vi "Read Data.vi"(8 "error in (no error)":errorcluster, 11 "WebSocket Data Handler Msg in":refnum<class "WebSocket Connection Handler Msg.lvclass">) -> (0 "error out":errorcluster, 2 "Data":string, 3 "WebSocket Data Handler Msg out":refnum<class "WebSocket Connection Handler Msg.lvclass">)   [LabVIEW 2016, in "WebSocket Actors.lvlib" / "WebSocket Connection Handler Msg.lvclass"]
uses:
  WebSocket Connection Handler Msg.lvclass
  WebSocket Connection Handler Msg.lvclass/WebSocket Connection Handler Msg.ctl
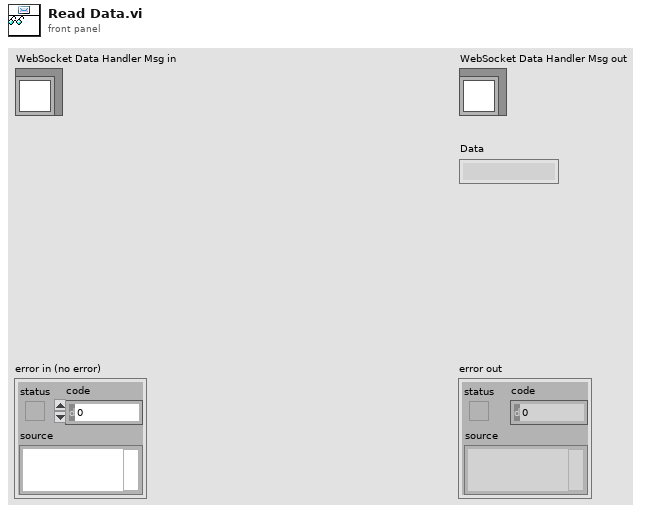
[diagram p1: front panel]
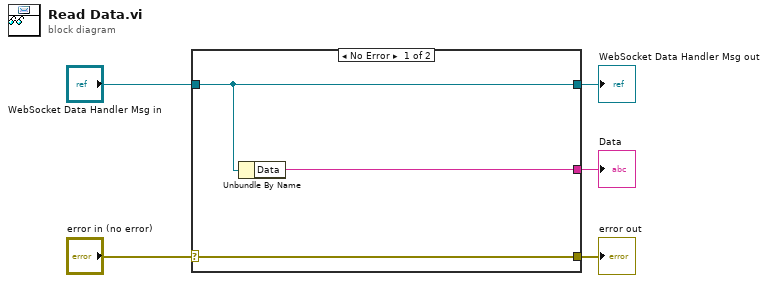
[diagram p0: block diagram]
diagram:
  n1 = case shown="No Error" "error in (no error)" {
    selector: "error in (no error)" -> [w8 w9]
    tunnel: [w8 w9] -> w4
    tunnel: [w7 w10] -> w2
    tunnel: "WebSocket Data Handler Msg in" -> [w7 w10]
    tunnel: [w6 _] -> w1
    frame No Error {
      n2 = Unbundle By Name(w7) -> ("Data"=w6:string)
    }
    frame Error {
    }
  }
  "error out" <- w4
  "WebSocket Data Handler Msg out" <- w2
  "Data" <- w1
